vi "Read Channel 2 U8 Array.vi"(8 "error in (no error)":errorcluster, 11 "Conversion in":refnum<class "Conversion.lvclass">) -> (0 "error out":errorcluster, 2 "Channel 2 U8 Array":u8[](array[numeric]), 3 "Conversion out":refnum<class "Conversion.lvclass">)   [LabVIEW 2023, in "Conversion.lvclass"]
uses:
  Conversion.lvclass
  Conversion.lvclass/Conversion.ctl
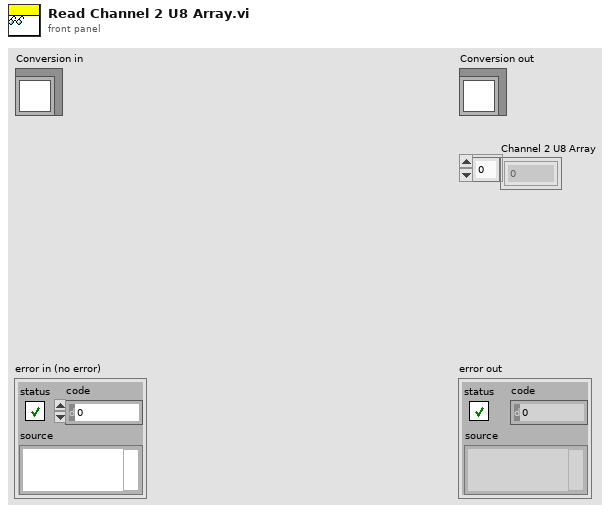
[diagram p1: front panel]
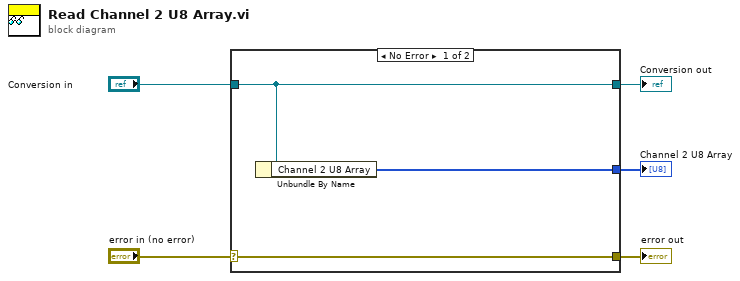
[diagram p0: block diagram]
diagram:
  n1 = case shown="No Error" "error in (no error)" {
    selector: "error in (no error)" -> [w8 w9]
    tunnel: [w8 w9] -> w4
    tunnel: [w7 w10] -> w2
    tunnel: "Conversion in" -> [w7 w10]
    tunnel: [w6 _] -> w1
    frame No Error {
      n2 = Unbundle By Name(w7) -> ("Channel 2 U8 Array"=w6:u8[])
    }
    frame Error {
    }
  }
  "error out" <- w4
  "Conversion out" <- w2
  "Channel 2 U8 Array" <- w1
